vi "Combine Operation.vi"(5 "initialize entry (F)":bool, 6 "chip select  (1st chip)":enum16{"1st chip", "2nd chip"}(ring), 7 "function set (F)":bool, 9 "cmd/data (0)":u8 format="%.0x", 10 "RS":bool, 11 "R/W":bool) -> (3 "output":u32 format="%.0x")   [LabVIEW 2015, in "HD44780 FPGA.lvlib"]
uses:
  <vilib>/EmbeddedDisplay/Hitachi HD44780/FPGA/HD44780 FPGA.lvlib
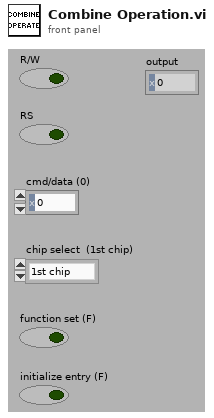
[diagram p1: front panel]
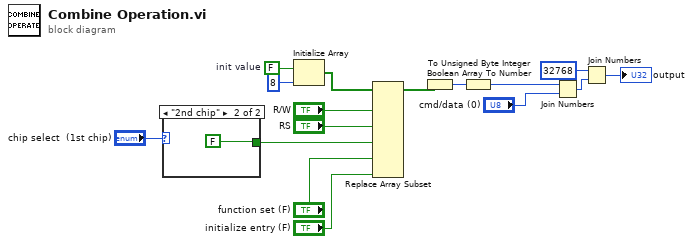
[diagram p0: block diagram]
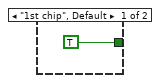
[diagram p2: hidden frame]
diagram:
  w9 = FALSE  # init value
  n1 = case shown="\"2nd chip\"" "chip select  (1st chip)" {
    tunnel: [TRUE FALSE] -> w5
    frame "1st chip", Default {
    }
    frame "2nd chip" {
    }
  }
  n2 = Initialize Array(w9, 8 ("dimension size")) -> (w1:bool[])
  n3 = Replace Array Subset(array=w1, new element #1="R/W", new element #2="RS", new element #3=w5, new element #4="function set (F)", new element #5="initialize entry (F)") -> (w2:bool[])  [unwired: 5 in]
  n4 = Boolean Array To Number(Boolean array=w2) -> (number=w14:u8)
  n5 = To Unsigned Byte Integer(number=w14) -> (unsigned 8bit integer=w13:u8)
  n6 = Join Numbers(hi=w13, lo="cmd/data (0)") -> ((hi.lo)=w12:u16)
  n7 = Join Numbers(hi=u16 32768, lo=w12) -> ((hi.lo)=→"output":u32)
